vi "resizeFrontPanel.vi"(8 "error in (no error)":errorcluster, 11 "PolymorphicInstance in":refnum<class "PolymorphicInstance.lvclass">) -> (0 "error out":errorcluster, 3 "PolymorphicInstance out":refnum<class "PolymorphicInstance.lvclass">)   [LabVIEW 2013, in "PolymorphicInstance.lvclass"]
uses:
  PolymorphicInstance.lvclass
  PolymorphicInstance.lvclass/PolymorphicInstance.ctl
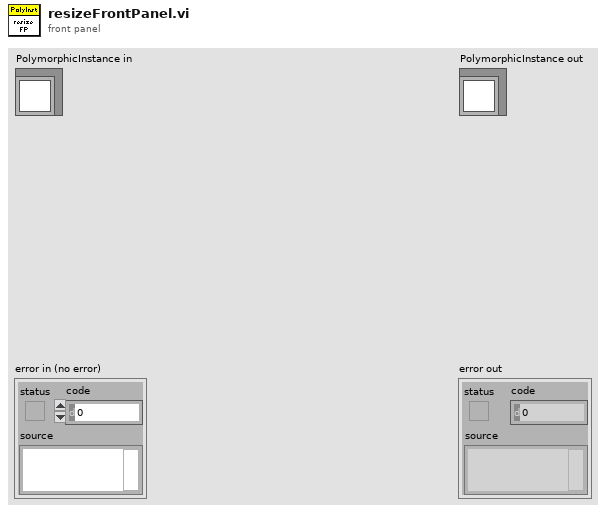
[diagram p1: front panel]
types:
  T1 = typedef "LVRectTypeDef.ctl" = cluster{"Left":i16, "Top":i16, "Right":i16, "Bottom":i16}
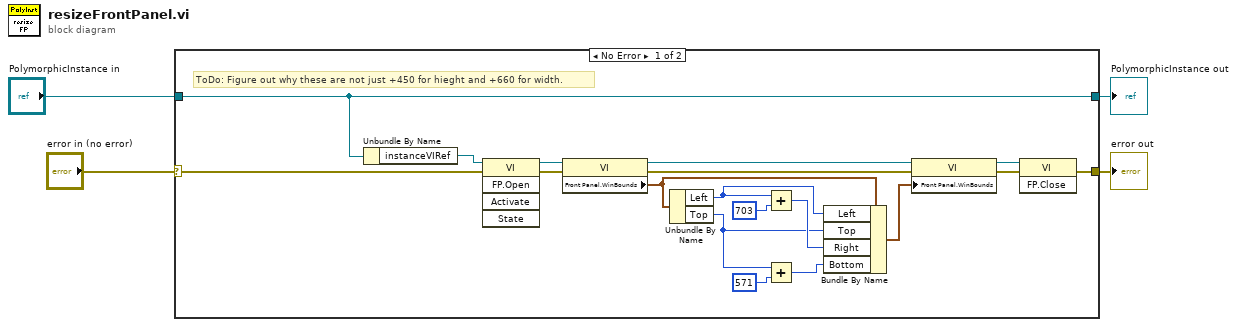
[diagram p0: block diagram]
diagram:
  n1 = case shown="No Error" "error in (no error)" {
    selector: "error in (no error)" -> [w18 w24]
    tunnel: [w17 w24] -> w3
    tunnel: [w22 w23] -> w1
    tunnel: "PolymorphicInstance in" -> [w22 w23]
    frame No Error {
      # "ToDo: Figure out why these are not just +450 for hieght and +660 for width."
      n2 = Unbundle By Name(w22) -> ("instanceVIRef"=w21:refnum<vi>)
      n3 = invoke class="VI" method="FP.Open"(reference=w21, error in=w18) -> (reference out=w20:refnum<vi>, error out=w19:errorcluster)  [unwired: 3 in, 3 out]
      n4 = property class="VI"(reference=w20, error in=w19) -> (reference out=w10:refnum<vi>, error out=w8:errorcluster, "Front Panel.WinBounds"=w16:T1)
      n5 = Unbundle By Name(w16) -> ("Left"=w14:i16, "Top"=w5:i16)
      n6 = Add(x=w14, y=i16 703) -> (x+y=w13:i16)
      n7 = Add(x=w5, y=i16 571 ("Left")) -> (x+y=w11:i16)
      n8 = Bundle By Name(cluster=w16, "Left"=w14, "Top"=w5, "Right"=w13, "Bottom"=w11) -> (w6:T1)
      n9 = property class="VI"(reference=w10, error in=w8, "Front Panel.WinBounds"=w6) -> (reference out=w9:refnum<vi>, error out=w7:errorcluster)
      n10 = invoke class="VI" method="FP.Close"(reference=w9, error in=w7) -> (error out=w17:errorcluster)  [unwired: 1 in, 2 out]
    }
    frame Error {
    }
  }
  "error out" <- w3
  "PolymorphicInstance out" <- w1
